vi "Get RPotRef.vi"(11 "arm in":refnum<class "arm.lvclass">) -> (2 "PotDevRef":T1={"DevStatus"={"status"=FALSE, "code"=0, "source"=""}, "Analog Channel"=enum."Invalid", "Invert Output"=FALSE}, 3 "arm out":refnum<class "arm.lvclass">)   [LabVIEW 2015, in "arm.lvclass"]
uses:
  arm.lvclass
  <vilib>/Rock Robotics/WPI/Potentiometer/WPI_PotentiometerDevRef.ctl
  <vilib>/Rock Robotics/SystemInterfaces/AI/FPGA_AIChannel.ctl
  arm.lvclass/arm.ctl
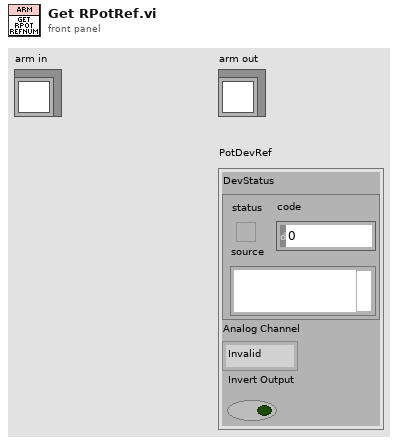
[diagram p1: front panel]
types:
  T1 = typedef "WPI_PotentiometerDevRef.ctl" = cluster{"DevStatus":errorcluster, "Analog Channel":T2, "Invert Output":bool}
  T2 = typedef "FPGA_AIChannel.ctl" = enum8{"AI 0", "AI 1", "AI 2", "AI 3", "AI MXP 0", "AI MXP 1", "AI MXP 2", "AI MXP 3", "Invalid"}
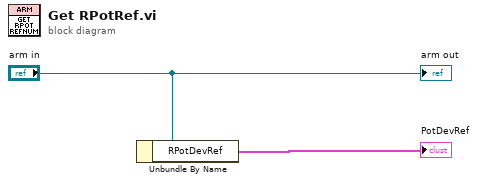
[diagram p0: block diagram]
diagram:
  n1 = Unbundle By Name("arm in") -> ("RPotDevRef"=→"PotDevRef":T1)
  "arm out" <- "arm in"
